vi "MQTT_Unsubscribe.vi"(8 "error in (no error)":errorcluster, 9 "Message ID":u16=10 format="%x", 10 "UnSubscribe Topic Array":string[](array[string]), 11 "SSL_Connection":T1) -> (0 "error out":errorcluster, 2 "Unsubscribe Message":u8[](array[numeric]) format="%x", 3 "SSL_Connection":T1)   [LabVIEW 2016, in "AWS_IoT.lvlib"]
doc: "This VI unsubscribes the client from a topic. The client can no longer read published messages for the topic. \n\n© 2015 - daq.io, LLC - Peter Adelhardt"
uses:
  AWS_IoT.lvlib
  Controls/SSL_Connection.ctl
  Controls/MessageType.ctl
  Controls/Retain_Flag.ctl
  Controls/DUP_Flag.ctl
  Controls/QoS.ctl
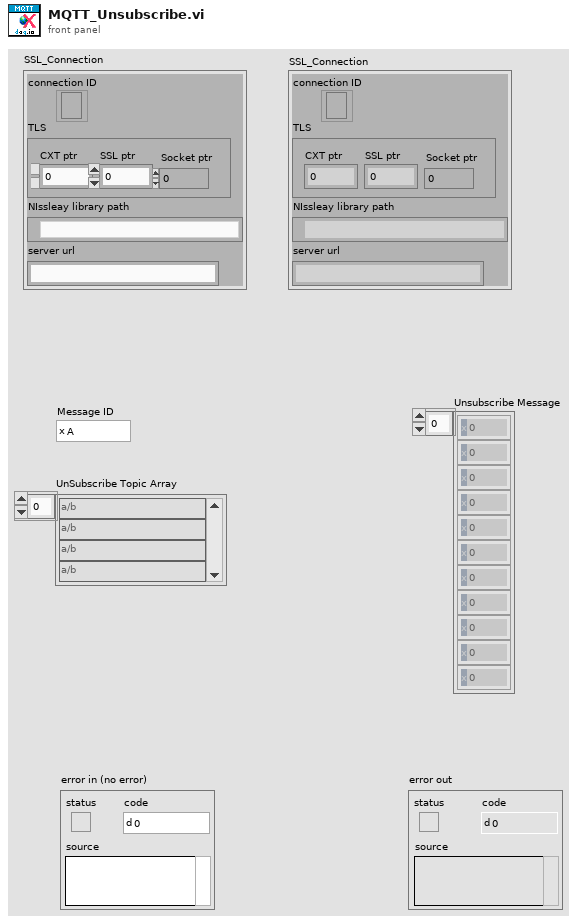
[diagram p1: front panel]
types:
  T1 = typedef "AWS_IoT.lvlib/SSL_Connection.ctl" = cluster{"connection ID":refnum<k5>, "TLS":cluster{"CXT ptr":i32, "SSL ptr":i32, "Socket ptr":i32}, "NIssleay library path":path, "server url":string}
  T2 = typedef "AWS_IoT.lvlib/QoS.ctl" = enum8{"At most once", "At least once", "Exactly once", "Reserved"}
  T3 = typedef "AWS_IoT.lvlib/DUP_Flag.ctl" = bool
  T4 = typedef "AWS_IoT.lvlib/Retain_Flag.ctl" = bool
  T5 = typedef "AWS_IoT.lvlib/MessageType.ctl" = enum32{"Reserved", "CONNECT", "CONNACK", "PUBLISH", "PUBACK", "PUBREC", "PUBREL", "PUBCOMP", "SUBSCRIBE", "SUBACK", "UNSUBSCRIBE", "UNSUBACK", "PINGREQ", "PINGRESP", "DISCONNECT", "Reserved2"}
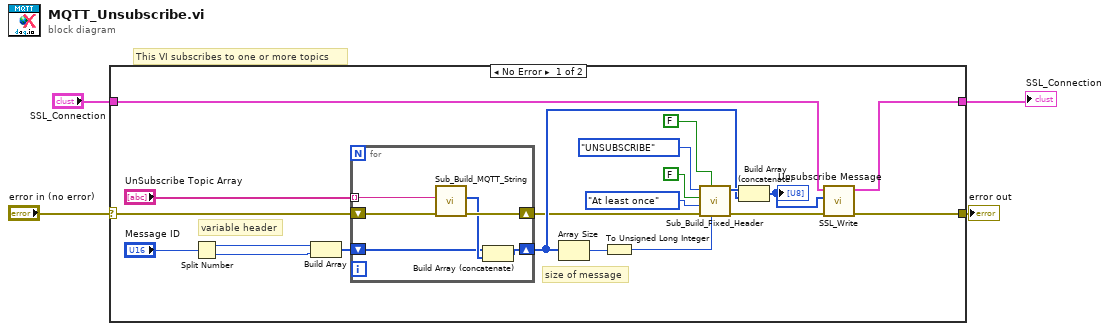
[diagram p0: block diagram]
diagram:
  # "This VI subscribes to one or more topics"
  n1 = case shown="No Error" "error in (no error)" {
    selector: "error in (no error)" -> [w17 w32]
    tunnel: [w8 w32] -> w3
    tunnel: "SSL_Connection" -> [w6 w31]
    tunnel: [w5 w31] -> w1
    frame No Error {
      # "variable header"
      # "size of message"
      n2 = Split Number(x="Message ID") -> (hi(x)=w20:u8, lo(x)=w19:u8)
      n3 = Build Array(w20, w19) -> (w14:u8[])
      n4 = for {
        tunnel: "UnSubscribe Topic Array" -> [w25] mode=indexing
        shift-right: [w29] -> w10
        shift-left: w17 -> [w30]
        shift-right: [w27] -> w16
        shift-left: w14 -> [w26]
        n5 = call "Sub_Build_MQTT_String.vi"("error in (no error)"=w30, "String to be encoded"=w25) -> ("error out"=w29:errorcluster, "UTF8 Byte Array"=w28:u8[])  [unwired: 8 in]
        n6 = Build Array (concatenate)(w26, w28) -> (w27:u8[])
      }
      n7 = Array Size(array=w16) -> (size(s)=w22:i32)
      n8 = To Unsigned Long Integer(number=w22) -> (unsigned 32bit integer=w23:u32)
      n9 = call "Sub_Build_Fixed_Header.vi"("Remaining Length"=w23, "Retain"=T4 FALSE, "error in (no error)"=w10, "QoS"=QoS."At least once", "DUP"=T3 FALSE, "MessageType"=MessageType."UNSUBSCRIBE") -> ("error out"=w9:errorcluster, "Fixed Header"=w21:u8[])  [unwired: 4 in]
      n10 = Build Array (concatenate)(w21, w16) -> (w7:u8[])
      "Unsubscribe Message" <- w7
      n11 = call "SSL_Write.vi"("error in (no error)"=w9, "data in"=w7, "SSL_Connection"=w6) -> ("error out"=w8:errorcluster, "SSL_Connection"=w5:T1)  [unwired: 7 in]
    }
    frame Error {
    }
  }
  "error out" <- w3
  "SSL_Connection" <- w1
